vi "moveToTargetPosition.vi"(1 "speed":dbl=2000.0 min=0.0 max=2000.0, 2 "Encoder COM Port":refnum<visa-resource-name>, 3 "targetPos":dbl, 4 "currentPos":dbl) -> (0 "updatedCurrentPos":dbl)   [LabVIEW 2013]
panel:
  # "The default motor speed is 2000 steps/second."
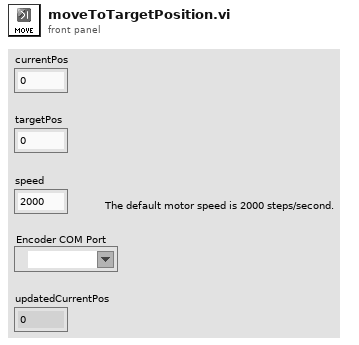
[diagram p1: front panel]
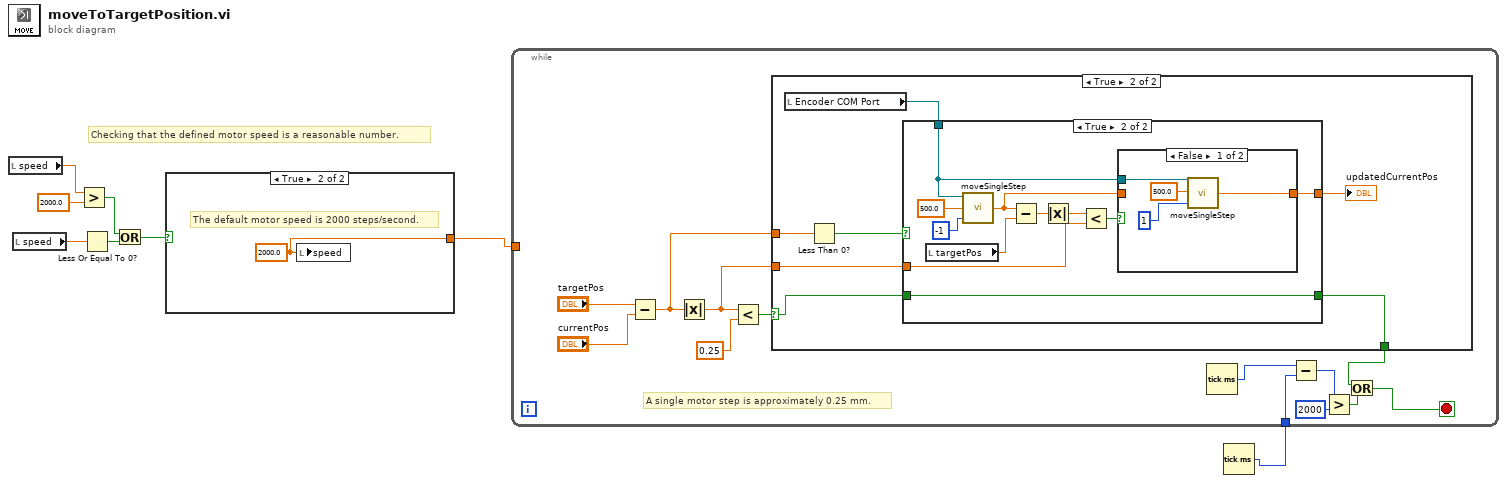
[diagram p0: block diagram]
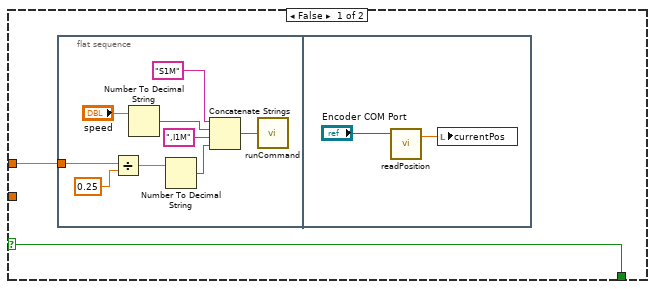
[diagram p3: hidden frame]
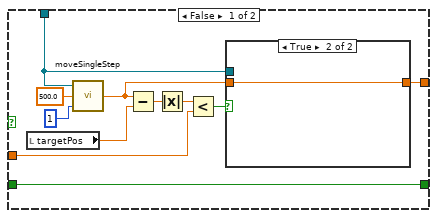
[diagram p4: hidden frame]
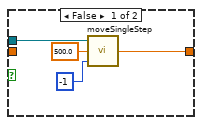
[diagram p5: hidden frame]
diagram:
  # "Checking that the defined motor speed is a reasonable number."
  n1 = local read "speed"() -> (w6:dbl)
  n2 = local read "speed"() -> (w3:dbl)
  n3 = Greater?(x=w6, y=2000.0) -> (0:w7:bool)
  n4 = Less Or Equal To 0?(x=w3) -> (x <= 0?=w5:bool)
  n5 = Or(x=w7, y=w5) -> (x .or. y?=w8:bool)
  n6 = case shown="True" w8 {
    tunnel: [_ w9] -> w2
    frame False {
    }
    frame True {
      w9 = 2000.0 ("speed")
      # "The default motor speed is 2000 steps/second."
      n7 = local write "speed"(w9) -> ()
    }
  }
  n8 = Tick Count (ms)() -> (millisecond timer value=w1:u32)
  n9 = while {
    tunnel: w2 -> [_]
    tunnel: w1 -> [w14]
    stop <- w10 stop-if-true
    # "A single motor step is approximately 0.25 mm."
    n10 = Subtract(x="targetPos", y="currentPos") -> (x-y=w19:dbl)
    n11 = Absolute Value(x=w19) -> (abs(x)=w17:dbl)
    n12 = Less?(x=w17, y=0.25) -> (x < y?=w20:bool)
    n13 = case shown="True" w20 {
      selector: w20 -> [w23 w38]
      tunnel: w19 -> [w24 w42]
      tunnel: w17 -> [_ w39]
      tunnel: [w23 w36] -> w16
      frame False {
        n14 = flat-sequence {
          tunnel: w24 -> [w31]
          frame #0 {
            n15 = Divide(x=w31, y=0.25) -> (x/y=w29:dbl)
            n16 = Number To Decimal String(number="speed") -> (decimal integer string=w26:string)  [unwired: 1 in]
            n17 = Number To Decimal String(number=w29) -> (decimal integer string=w33:string)  [unwired: 1 in]
            n18 = Concatenate Strings("S1M" ("string"), w26, ",I1M" ("string"), w33) -> (w32:string)
            n19 = call "runCommand.vi"("command"=w32) -> ()  [unwired: 1 in]
          }
          frame #1 {
            n20 = call "readPosition.vi"("VISA resource name"="Encoder COM Port") -> ("position"=w35:dbl)  [unwired: 1 in, 2 out]
            n21 = local write "currentPos"(w35) -> ()
          }
        }
      }
      frame True {
        n22 = local read "Encoder COM Port"() -> (w40:refnum<visa-resource-name>)
        n23 = Less Than 0?(x=w42) -> (x < 0?=w41:bool)
        n24 = case shown="True" w41 {
          tunnel: w40 -> [w46 w63]
          tunnel: w39 -> [w47 w64]
          tunnel: w38 -> [w44 w60]
          tunnel: [w45 w61] -> w37
          tunnel: [w44 w60] -> w36
          frame False {
            n25 = local read "targetPos"() -> (w49:dbl)
            n26 = call "moveSingleStep.vi"("direction"=1, "motorSpeed"=500.0, "VISA resource name"=w46) -> ("position"=w53:dbl)
            n27 = Subtract(x=w53, y=w49) -> (x-y=w50:dbl)
            n28 = Absolute Value(x=w50) -> (abs(x)=w51:dbl)
            n29 = Less?(x=w51, y=w47) -> (x < y?=w52:bool)
            n30 = case shown="True" w52 {
              tunnel: w53 -> [_ w58]
              tunnel: w46 -> [w56 _]
              tunnel: [w55 w58] -> w45
              frame False {
                n31 = call "moveSingleStep.vi"("direction"=-1, "motorSpeed"=500.0, "VISA resource name"=w56) -> ("position"=w55:dbl)
              }
              frame True {
              }
            }
          }
          frame True {
            n32 = local read "targetPos"() -> (w68:dbl)
            n33 = call "moveSingleStep.vi"("direction"=-1, "motorSpeed"=500.0, "VISA resource name"=w63) -> ("position"=w62:dbl)
            n34 = Subtract(x=w62, y=w68) -> (x-y=w67:dbl)
            n35 = Absolute Value(x=w67) -> (abs(x)=w65:dbl)
            n36 = Less?(x=w65, y=w64) -> (x < y?=w66:bool)
            n37 = case shown="False" w66 {
              tunnel: w63 -> [w73 _]
              tunnel: w62 -> [_ w74]
              tunnel: [w71 w74] -> w61
              frame False {
                n38 = call "moveSingleStep.vi"("direction"=1, "motorSpeed"=500.0, "VISA resource name"=w73) -> ("position"=w71:dbl)
              }
              frame True {
              }
            }
          }
        }
        "updatedCurrentPos" <- w37
      }
    }
    n39 = Tick Count (ms)() -> (millisecond timer value=w15:u32)
    n40 = Subtract(x=w15, y=w14) -> (x-y=w13:u32)
    n41 = Greater?(x=w13, y=u32 2000) -> (0:w11:bool)
    n42 = Or(x=w16, y=w11) -> (x .or. y?=w10:bool)
  }
